vi "Bytes at port more eq 0 or less X.vi"(0 "X":u32, 1 "serial ref  name":refnum<visa-resource-name>, 5 "error IO":errorcluster) -> (9 "Bytes at port <X or = 0?":bool, 14 "serial out":refnum<visa-resource-name>, 16 "Num. of Bytes at Port":u32, 19 "error out":errorcluster)   [LabVIEW 2013]
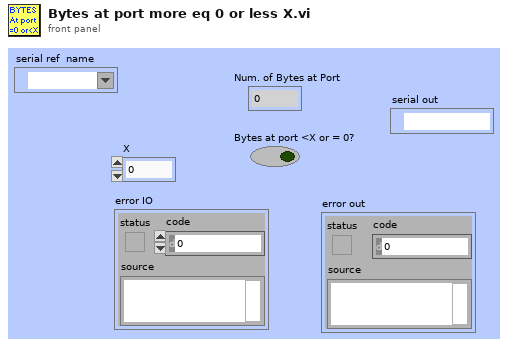
[diagram p1: front panel]
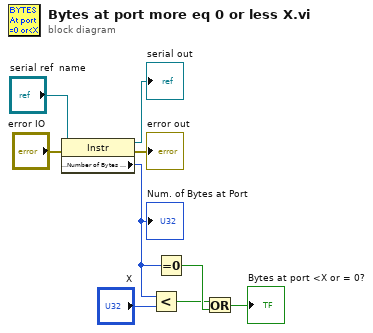
[diagram p0: block diagram]
diagram:
  n1 = property class="Instr"(reference="serial ref  name", error in="error IO") -> (reference out=→"serial out":refnum<visa-resource-name>, error out=→"error out":errorcluster, "Serial Settings:Number of Bytes at Serial Port"=w5:u32)
  "Num. of Bytes at Port" <- w5
  n2 = Less?(x=w5, y="X") -> (x < y?=w3:bool)
  n3 = Equal To 0?(x=w5) -> (x = 0?=w4:bool)
  n4 = Or(x=w3, y=w4) -> (x .or. y?=→"Bytes at port <X or = 0?":bool)
